vi "Analyze Waveforms.vi"(5 "Waveform Array Chart Ref":refnum<vi>) -> ()   [LabVIEW 2012]
panel:
  in  "Exit":bool
  in  "Reset Scale":bool
  in  "Log Info Button":bool
  in  "Snapshot":bool
  in  "Open Log":bool
  in  "Rescale Y":bool
  out "Cursor Delta (T2 - T1)":cluster{"X":dbl, "Y":dbl, "Y 2":dbl} {"Y 2" format="%9.3p"; "Y" format="%9.3p"; "X" format="%.3g"}
  out "Cursor T2":cluster{"X":dbl, "Y":dbl, "Y 2":dbl} {"Y 2" format="%9.3p"; "Y" format="%9.3p"; "X" format="%.3g"}
  out "Cursor T1":cluster{"X":dbl, "Y":dbl, "Y 2":dbl} {"Y 2" format="%9.3p"; "Y" format="%9.3p"; "X" format="%.3g"}
  out "Analyze Signals":waveform(dbl)[](graph)
  # "Analyze Waveform Signals"
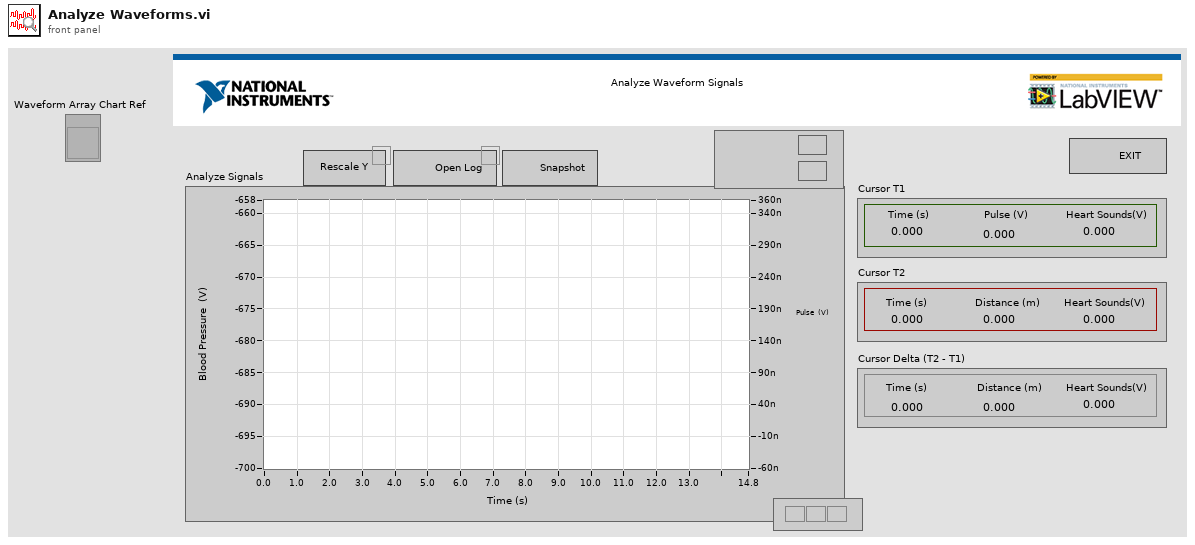
[diagram p1: front panel]
types:
  T1 = typedef "LVRangeTypeDef.ctl" = cluster{"Minimum":dbl, "Maximum":dbl, "Increment":dbl, "Minor Increment":dbl, "Start":dbl}
  T2 = cluster{"Cursor.Cursor X":dbl, "Cursor.Cursor Y":dbl, dbl}
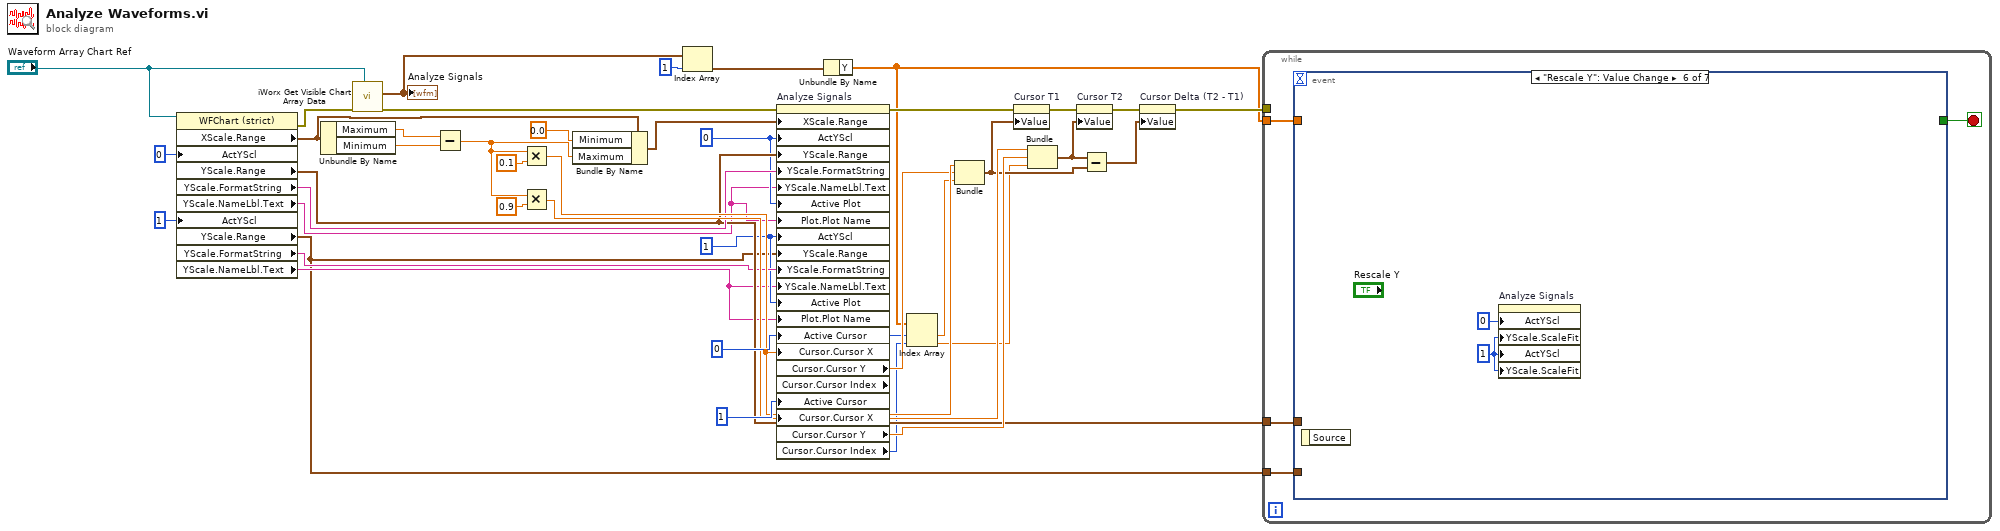
[diagram p0: block diagram]
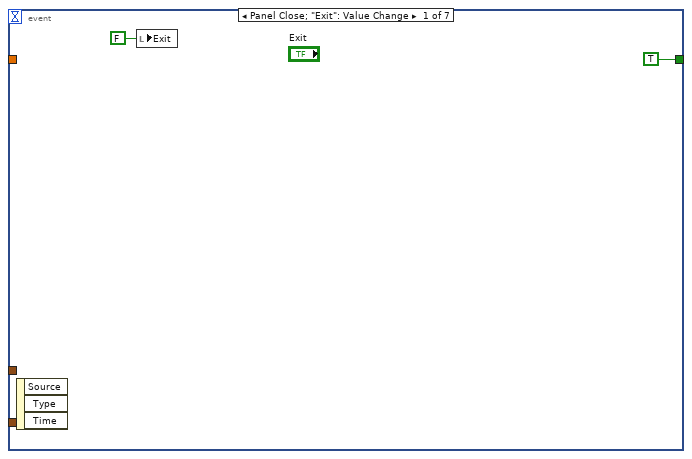
[diagram p2: hidden frame]
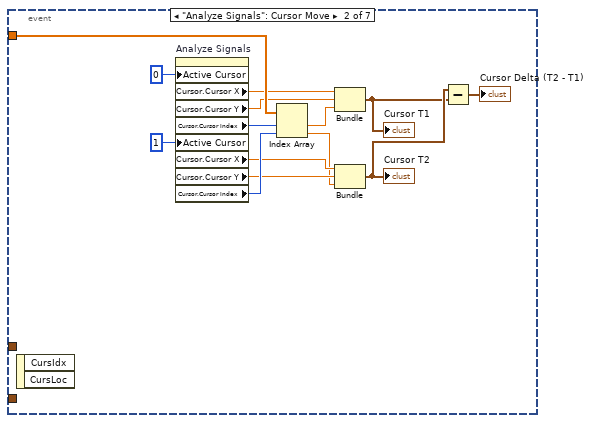
[diagram p3: hidden frame]
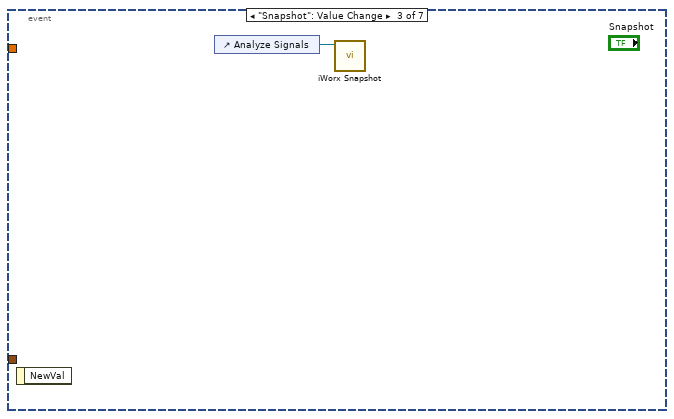
[diagram p4: hidden frame]
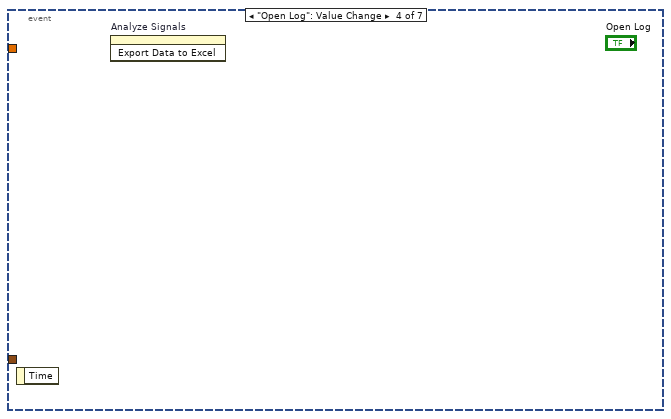
[diagram p5: hidden frame]
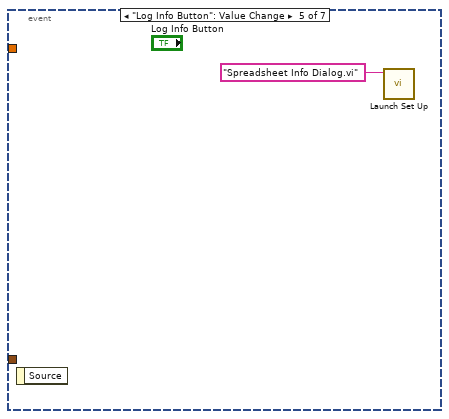
[diagram p6: hidden frame]
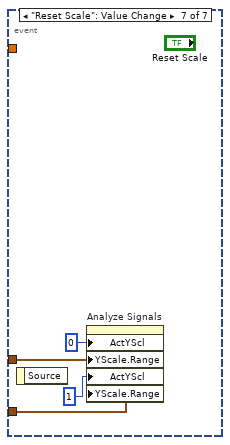
[diagram p7: hidden frame]
diagram:
  w5 = 1 ("Active Y Scale")
  w3 = 0 ("Active Y Scale")
  n1 = property on="Property Node" class="WFChart (strict)"(reference="Waveform Array Chart Ref", "ActYScl"=0 ("Active Y Scale"), "ActYScl"=1 ("Active Y Scale")) -> (error out=w17:errorcluster, "XScale.Range"=w40:T1, "YScale.Range"=w22:T1, "YScale.FormatString"=w23:string, "YScale.NameLbl.Text"=w2:string, "YScale.Range"=w1:T1, "YScale.FormatString"=w18:string, "YScale.NameLbl.Text"=w4:string)  [unwired: 1 in, 1 out]
  n2 = Unbundle By Name(w40) -> ("Maximum"=w42:dbl, "Minimum"=w41:dbl)
  n3 = call "iWorx Get Visible Chart Array Data.vi"("Waveform Chart 3"="Waveform Array Chart Ref", "Error In"=w17) -> ("Error Out"=w16:errorcluster, "Waveforms Out"=w14:waveform(dbl)[])  [unwired: 8 in]
  "Analyze Signals" <- w14
  n4 = Subtract(x=w42, y=w41) -> (x-y=w33:dbl)
  n5 = Multiply(x=w33, y=0.1) -> (x*y=w32:dbl)
  n6 = Multiply(x=w33, y=0.9) -> (x*y=w29:dbl)
  n7 = Bundle By Name(cluster=w40, "Minimum"=0.0, "Maximum"=w33) -> (w38:T1)
  n8 = Index Array(array=w14, index=1) -> (element=w11:waveform(dbl))
  n9 = property on="Analyze Signals" class="WFGraph (strict)"(error in=w16, "XScale.Range"=w38, "ActYScl"=w3, "YScale.Range"=w22, "YScale.FormatString"=w23, "YScale.NameLbl.Text"=w2, "Active Plot"=w3, "Plot.Plot Name"=w2, "ActYScl"=w5, "YScale.Range"=w1, "YScale.FormatString"=w18, "YScale.NameLbl.Text"=w4, "Active Plot"=w5, "Plot.Plot Name"=w4, "Active Cursor"=u32 0, "Cursor.Cursor X"=w32, "Active Cursor"=u32 1, "Cursor.Cursor X"=w29) -> (error out=w15:errorcluster, "Cursor.Cursor Y"=w31:dbl, "Cursor.Cursor Index"=w10:i32, "Cursor.Cursor Y"=w28:dbl, "Cursor.Cursor Index"=w9:i32)  [unwired: 1 in, 1 out]
  n10 = Unbundle By Name(w11) -> ("Y"=w6:dbl[])
  n11 = Index Array(array=w6, index #1=w10, index #2=w9) -> (element #1=w8:dbl, element #2=w7:dbl)
  n12 = Bundle(w32, "Cursor.Cursor Y"=w31, w8) -> (w26:cluster{dbl, "Cursor.Cursor Y":dbl, dbl})  [unwired: 1 in]
  n13 = property on="Cursor T1" class="Clust (strict)"(error in=w15, "Value"=w26) -> (error out=w30:errorcluster)  [unwired: 1 in, 1 out]
  n14 = Bundle(w29, "Cursor.Cursor Y"=w28, w7) -> (w27:cluster{dbl, "Cursor.Cursor Y":dbl, dbl})  [unwired: 1 in]
  n15 = property on="Cursor T2" class="Clust (strict)"(error in=w30, "Value"=w27) -> (error out=w25:errorcluster)  [unwired: 1 in, 1 out]
  n16 = Subtract(x=w27, y=w26) -> (x-y=w24:cluster{dbl, "Cursor.Cursor Y":dbl, dbl})
  n17 = property on="Cursor Delta (T2 - T1)" class="Clust (strict)"(error in=w25, "Value"=w24) -> (error out=w12:errorcluster)  [unwired: 1 in, 1 out]
  n18 = while {
    tunnel: w22 -> [w45]
    tunnel: w12 -> [_]
    tunnel: w6 -> [w44]
    tunnel: w1 -> [w43]
    stop <- w46 stop-if-true
    n19 = event shown="[5] \"Rescale Y\": Value Change" {
      selector: _ -> [_ _ _ _ _ _ _]
      dyn-events: _ -> [_ _ _ _ _ _ _]
      timeout: _ -> [_ _ _ _ _ _ _]
      tunnel: [TRUE _ _ _ _ _ _] -> w46
      tunnel: w45 -> [_ _ _ _ _ _ w70]
      tunnel: w44 -> [_ w58 _ _ _ _ _]
      tunnel: w43 -> [_ _ _ _ _ _ w67]
      event Panel Close; "Exit": Value Change {
        n20 = event-data() -> ()  [unwired: 1 in, 3 out]
        n21 = local write "Exit"(FALSE ("Exit")) -> ()
      }
      event "Analyze Signals": Cursor Move {
        n22 = event-data() -> ()  [unwired: 1 in, 2 out]
        n23 = property on="Analyze Signals" class="WFGraph (strict)"("Active Cursor"=u32 0, "Active Cursor"=u32 1) -> ("Cursor.Cursor X"=w57:dbl, "Cursor.Cursor Y"=w56:dbl, "Cursor.Cursor Index"=w60:i32, "Cursor.Cursor X"=w54:dbl, "Cursor.Cursor Y"=w53:dbl, "Cursor.Cursor Index"=w59:i32)  [unwired: 2 in, 2 out]
        n24 = Index Array(array=w58, index #1=w60, index #2=w59) -> (element #1=w55:dbl, element #2=w52:dbl)
        n25 = Bundle("Cursor.Cursor X"=w57, "Cursor.Cursor Y"=w56, w55) -> (w50:T2)  [unwired: 1 in]
        "Cursor T1" <- w50
        n26 = Bundle("Cursor.Cursor X"=w54, "Cursor.Cursor Y"=w53, w52) -> (w51:T2)  [unwired: 1 in]
        "Cursor T2" <- w51
        n27 = Subtract(x=w51, y=w50) -> (x-y=→"Cursor Delta (T2 - T1)":T2)
      }
      event "Snapshot": Value Change {
        n28 = event-data() -> ()  [unwired: 1 in, 1 out]
        n29 = control-ref of="Analyze Signals"() -> (w63:refnum<vi>)
        n30 = call "iWorx Snapshot.vi"("WaveformChart in"=w63) -> ()  [unwired: 10 in, 1 out]
      }
      event "Open Log": Value Change {
        n31 = event-data() -> ()  [unwired: 1 in, 1 out]
        n32 = invoke on="Analyze Signals" class="WFGraph (strict)" method="Export Data to Excel"() -> ()  [unwired: 3 in, 3 out]
      }
      event "Log Info Button": Value Change {
        n33 = event-data() -> ()  [unwired: 1 in, 1 out]
        n34 = call "Launch Set Up.vi"("name or relative path"="Spreadsheet Info Dialog.vi") -> ()  [unwired: 9 in, 2 out]
      }
      event "Rescale Y": Value Change {
        w65 = 1 ("Active Y Scale")
        n35 = event-data() -> ()  [unwired: 1 in, 1 out]
        n36 = property on="Analyze Signals" class="WFGraph (strict)"("ActYScl"=0 ("Active Y Scale"), "YScale.ScaleFit"=w65, "ActYScl"=w65, "YScale.ScaleFit"=w65) -> ()  [unwired: 2 in, 2 out]
      }
      event "Reset Scale": Value Change {
        n37 = event-data() -> ()  [unwired: 1 in, 1 out]
        n38 = property on="Analyze Signals" class="WFGraph (strict)"("ActYScl"=0 ("Active Y Scale"), "YScale.Range"=w70, "ActYScl"=1 ("Active Y Scale"), "YScale.Range"=w67) -> ()  [unwired: 2 in, 2 out]
      }
    }
  }
